vi "Initialize.vi"(8 "error in (no error)":errorcluster, 9 "Reset (True)":bool=TRUE, 10 "ID Query (True)":bool=TRUE, 11 "VISA resource name":refnum<visa-resource-name>) -> (0 "error out":errorcluster, 3 "VISA resource name out":refnum<visa-resource-name>)   [LabVIEW 2018, in "Agilent MXA Series.lvlib"]
doc: "Establishes communication with the instrument and optionally performs an instrument identification query and/or an instrument reset. It also places the instrument in a default state needed for other instrument driver operations. Therefore, call this VI before calling other instrument driver VIs for this instrument. Generally, you need to call the Initialize VI only once at the beginning of an application."
uses:
  Agilent MXA Series.lvlib
  Private/Extended User Data.ctl
  <vilib>/regexp/Match Regular Expression.xnode
panel:
  # "(c) 2007-2015 National Instruments.  ALL RIGHTS RESERVED."
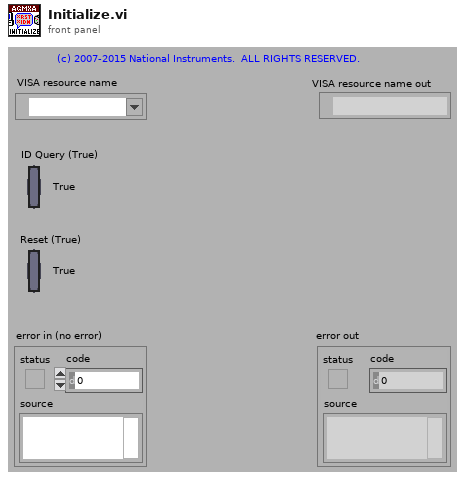
[diagram p1: front panel]
types:
  T1 = typedef "Agilent MXA Series.lvlib/Extended User Data.ctl" = cluster{"Measurement Type":i32, "Agilent MXA/EXA Model":i32}
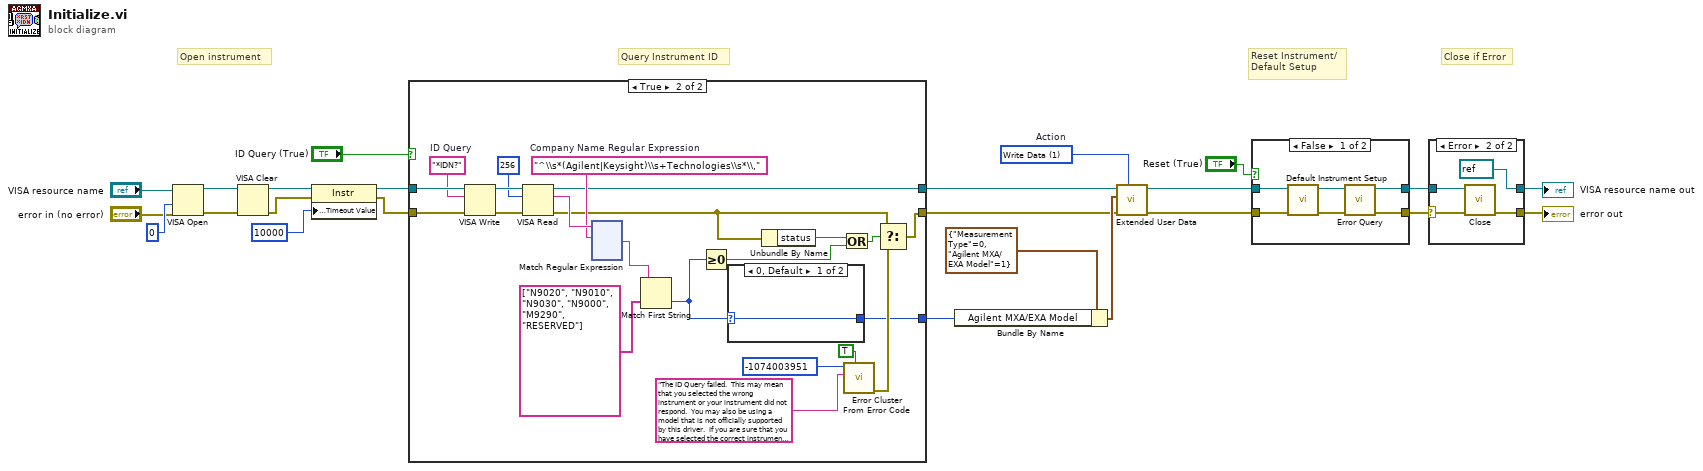
[diagram p0: block diagram]
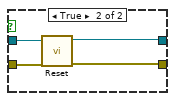
[diagram p3: hidden frame]
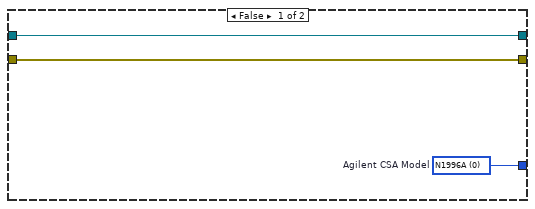
[diagram p4: hidden frame]
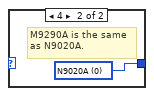
[diagram p5: hidden frame]
diagram:
  w1 = 1 items=["Read Data", "Write Data", "Clear Data", "Clear ALL Data"]  # Action
  # "Close if Error"
  # "Query Instrument ID"
  # "Reset Instrument/\nDefault Setup"
  # "Open instrument"
  n1 = VISA Open(access mode=u32 0, error in (no error)="error in (no error)", VISA resource name="VISA resource name") -> (VISA resource name=w15:refnum<visa-resource-name>, error out=w14:errorcluster)  [unwired: 2 in]
  n2 = VISA Clear(VISA resource name=w15, error in (no error)=w14) -> (VISA resource name out=w13:refnum<visa-resource-name>, error out=w12:errorcluster)
  n3 = property class="Instr"(reference=w13, error in=w12, "General Settings:Timeout Value"=u32 10000) -> (reference out=w17:refnum<visa-resource-name>, error out=w18:errorcluster)
  n4 = case shown="True" "ID Query (True)" {
    tunnel: [w26 w49] -> w4
    tunnel: [w27 w31] -> w5
    tunnel: w17 -> [w27 w47]
    tunnel: w18 -> [w26 w48]
    tunnel: [w25 w28] -> w16
    frame False {
      w25 = u16 0 items=["N1996A"]  # Agilent CSA Model
    }
    frame True {
      w33 = "^\\s*(Agilent|Keysight)\\s+Technologies\\s*\\,"  # Company Name Regular Expression
      w43 = "*IDN?"  # ID Query
      n5 = VISA Write(VISA resource name=w47, write buffer=w43, error in (no error)=w48) -> (VISA resource name out=w46:refnum<visa-resource-name>, error out=w45:errorcluster)  [unwired: 1 out]
      n6 = VISA Read(VISA resource name=w46, byte count=u32 256, error in (no error)=w45) -> (VISA resource name out=w31:refnum<visa-resource-name>, read buffer=w34:string, error out=w30:errorcluster)  [unwired: 1 out]
      n7 = xnode "Match Regular Expression"("input string"=w34, "regular expression"=w33) -> ("after match"=w32:string)  [unwired: 4 in, 4 out]
      n8 = Match First String(2:string[] ["N9020", "N9010", "N9030", "N9000", "M9290", "RESERVED"], 3:w32) -> (0:w29:i32)  [unwired: 1 out]
      n9 = Greater Or Equal To 0?(x=w29) -> (x >= 0?=w37:bool)
      n10 = case shown="0, Default" w29 {
        selector: w29 -> [w50 _]
        tunnel: [w50 w51] -> w28
        frame 0, Default {
        }
        frame 4 {
          w51 = 0 items=["N9020A", "N9010A", "N9030A", "N9000A"] ("Agilent MXA/EXA Model")
          # "M9290A is the same\nas N9020A."
        }
      }
      n11 = Unbundle By Name(w30) -> ("status"=w38:bool)
      n12 = Or(x=w38, y=w37) -> (x .or. y?=w36:bool)
      n13 = call <vilib>:"Error Cluster From Error Code.vi"("show call chain? (False)"=TRUE, "error message (\"\")"="The ID Query failed.  This may mean that you selected the wrong instrument or your instrument did not respond.  You may also be using a model that is not officially supported by this driver.  If you are sure that you have selected the correct instrument and it is responding, try disabling the ID Query." ("Source (VI Name)"), "error code (0)"=-1074003951 ("Code")) -> ("error out"=w42:errorcluster)  [unwired: 6 in]
      n14 = Select(t=w30, s=w36, f=w42) -> (s? t:f=w49:errorcluster)
    }
  }
  n15 = Bundle By Name(cluster=T1 {"Measurement Type"=0, "Agilent MXA/EXA Model"=1} ("User Data In"), "Agilent MXA/EXA Model"=w16) -> (w6:T1)
  n16 = call "Extended User Data.vi"("Action (1:Write Data)"=w1, "Error In (no error)"=w4, "User Data In"=w6, "VISA resource name in"=w5) -> ("Error Out"=w2:errorcluster, "VISA resource name out"=w3:refnum<visa-resource-name>)  [unwired: 5 in, 1 out]
  n17 = case shown="False" "Reset (True)" {
    tunnel: w2 -> [w167 w170]
    tunnel: [w163 w169] -> w19
    tunnel: w3 -> [w168 w171]
    tunnel: [w166 w172] -> w20
    frame False {
      n18 = call "Default Instrument Setup.vi"("error in (no error)"=w167, "VISA resource name"=w168) -> ("error out"=w164:errorcluster, "VISA resource name out"=w165:refnum<visa-resource-name>)  [unwired: 8 in]
      n19 = call "Error Query.vi"("error in (no error)"=w164, "VISA resource name"=w165) -> ("error out"=w163:errorcluster, "VISA resource name out"=w166:refnum<visa-resource-name>)  [unwired: 6 in, 2 out]
    }
    frame True {
      n20 = call "Reset.vi"("error in (no error)"=w170, "VISA resource name"=w171) -> ("error out"=w169:errorcluster, "VISA resource name out"=w172:refnum<visa-resource-name>)  [unwired: 8 in]
    }
  }
  n21 = case shown="Error" w19 {
    selector: w19 -> [w173 w175]
    tunnel: w20 -> [w174 w176]
    tunnel: [w174 refnum<visa-resource-name> refnum ("VISA resource name out")] -> w9
    tunnel: [w173 w177] -> w8
    frame No Error {
    }
    frame Error {
      n22 = call "Close.vi"("error in (no error)"=w175, "VISA resource name"=w176) -> ("error out"=w177:errorcluster)  [unwired: 9 in]
    }
  }
  "VISA resource name out" <- w9
  "error out" <- w8
